vi "Accelerometer Config Pane.vi"(6 "_SubPanelMessages":refnum<notifier>, 9 "_myEmbeddedToFrameEvent":T6, 10 "_myEmbedded.Exit":refnum<user-event>, 11 "_Property Bundle":cluster{"Name":string, "Value":variant}[](array[cluster])) -> (1 "_Connection Informations":T1, 2 "_Scripter Input":T8)   [LabVIEW 2021]
doc: "Reads acceleration values along the X, Y, and Z axes of the accelerometer on the NI myRIO."
uses:
  <vilib>/myRIO/Common/Express VI Framework/typedefs/Config Pane to Framework Ref.ctl
  <vilib>/myRIO/Common/Express VI Framework/typedefs/Data Validate Ref.ctl
  <vilib>/myRIO/Common/Express VI Framework/typedefs/Scripter Input.ctl
  <vilib>/myRIO/Common/Express VI Framework/typedefs/WireThrough Terminal Names.ctl
  <vilib>/myRIO/Common/Express VI Framework/typedefs/Instrument Driver Method Descriptor Array.ctl
  <vilib>/myRIO/Common/Express VI Framework/typedefs/Instrument Driver Method Descriptor.ctl
  <vilib>/myRIO/Common/Express VI Framework/typedefs/Sub Panel Messages.ctl
  <vilib>/myRIO/Express VI/Onboard Devices/Accelerometer/Accelerometer Images.ctl
  <vilib>/myRIO/Common/Express VI Framework/typedefs/Connection Informations.ctl
  <vilib>/myRIO/Common/Instrument Driver Framework/Utilities/typedefs/Channel Types.ctl
  <vilib>/myRIO/Common/Express VI Framework/vis/Express VI Framework Strings Global.vi
panel:
  out "_AccelerometerAxes":T2
  in  "Z Axis Custom Terminal Name":string
  in  "Z Enable":bool=TRUE
  in  "Y Axis Custom Terminal Name":string
  in  "Y Enable":bool=TRUE
  in  "X Axis Custom Terminal Name":string
  in  "X Enable":bool=TRUE
  in  "_Default Alias String":string
  in  "_VI Default Name (Edit and make value default)":string="Accelerometer"
  in  "Name:":string caption="Node name:"
  in  "_WireThrough Info (Edit and make value default)":T3={"WireThrough Top In"="Accelerometer Ref In", "WireThrough Bottom In"="error in (no error)", "WireThrough Top Out"="Accelerometer Ref Out", "WireThrough Bottom Out"="error out"}
  in  "_Template Array (Edit and make value default)":T4=[{"Function Name"="Smart Open", "VI Path"=path "<vilib>/myRIO/Instrument Drivers/Onboard Devices/Accelerometer/vis", "Script"=TRUE, "Inputs"=[{"name"="Channel Names", "value"=variant, "Config Pane Only"=TRUE, "Build Array"=FALSE, "Bundle Cluster"=FALSE, "Show Term"=FALSE, "alias"=[], "Required Input"=FALSE}], "Outputs"=[], "VI Class"=enum."Open", "Controls Refs[]"=[], "Inline"=FALSE}, {"Function Name"="Open", "VI Path"=path "<vilib>/myRIO/Instrument Drivers/Onboard Devices/Accelerometer/vis", "Script"=FALSE, "Inputs"=[], "Outputs"=[{"name"="Values", "value"=variant, "Show Term"=TRUE, "Index Array"=TRUE, "Unbundle Cluster"=FALSE, "alias"=["AccelerationX", "AccelerationY", "AccelerationZ"]}], "VI Class"=enum."Open", "Controls Refs[]"=[], "Inline"=FALSE}, {"Function Name"="Read", "VI Path"=path "<vilib>/myRIO/Instrument Drivers/Onboard Devices/Accelerometer/vis", "Script"=TRUE, "Inputs"=[], "Outputs"=[{"name"="Values", "value"=variant, "Show Term"=TRUE, "Index Array"=TRUE, "Unbundle Cluster"=FALSE, "alias"=["AccelerationX", "AccelerationY", "AccelerationZ"]}], "VI Class"=enum."Data", "Controls Refs[]"=[], "Inline"=FALSE}, {"Function Name"="Close", "VI Path"=path "<vilib>/myRIO/Instrument Drivers/Onboard Devices/Accelerometer/vis", "Script"=FALSE, "Inputs"=[], "Outputs"=[], "VI Class"=enum."Close", "Controls Refs[]"=[], "Inline"=FALSE}]
  in  "_Test Close":bool
  # "Range determines the sensitivity of the accelerometer."
  # "User Visible Area"
  # "Enable:"
  # "Custom channel name:"
  # "NOTE: Tab Order has been set\nfor this Front Panel.\n\nSee Edit>>Set Tabbing Order...\n\nAll controls that are not visible at \nruntime are excluded from Tabbing order\n\nTo exlude a control from context\nhelp prefix its label text with a '-'"
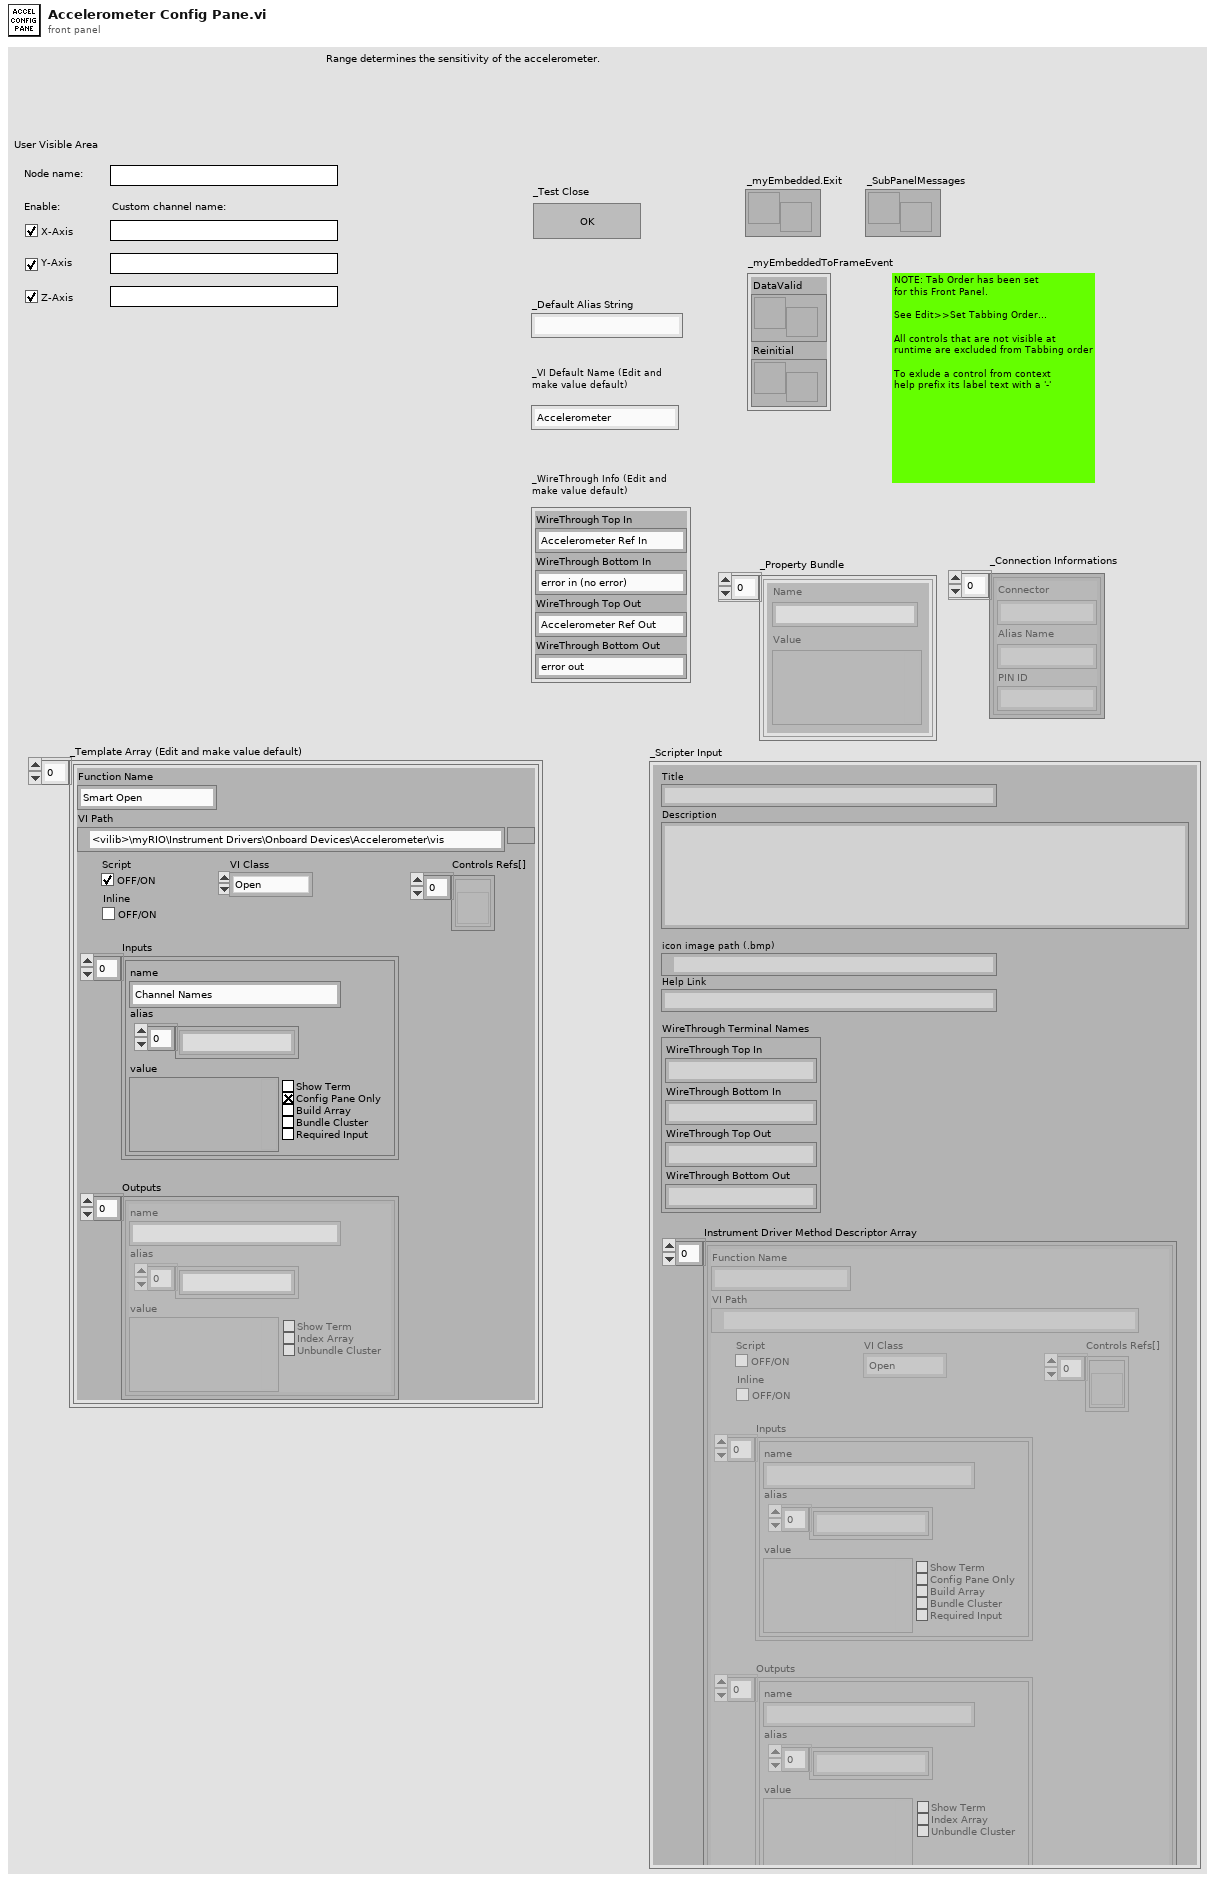
[diagram p1: front panel]
types:
  T1 = typedef "Connection Informations.ctl" = cluster{"Connector":string, "Alias Name":string, "PIN ID":string}[]
  T2 = typedef "Accelerometer Images.ctl" = u16
  T3 = typedef "WireThrough Terminal Names.ctl" = cluster{"WireThrough Top In":string, "WireThrough Bottom In":string, "WireThrough Top Out":string, "WireThrough Bottom Out":string}
  T4 = typedef "Instrument Driver Method Descriptor Array.ctl" = T5[]
  T5 = typedef "Instrument Driver Method Descriptor.ctl" = cluster{"Function Name":string, "VI Path":path, "Script":bool, "Inputs":cluster{"name":string, "value":variant, "Config Pane Only":bool, "Build Array":bool, "Bundle Cluster":bool, "Show Term":bool, "alias":string[], "Required Input":bool}[], "Outputs":cluster{"name":string, "value":variant, "Show Term":bool, "Index Array":bool, "Unbundle Cluster":bool, "alias":string[]}[], "VI Class":enum16{"Open", "Configure", "Data", "Manage", "Close"}, "Controls Refs[]":refnum<vi>[], "Inline":bool}
  T6 = typedef "Config Pane to Framework Ref.ctl" = cluster{"DataValid":T7, "Reinitial":refnum<user-event>}
  T7 = typedef "Data Validate Ref.ctl" = refnum<user-event>
  T8 = typedef "Scripter Input.ctl" = cluster{"Title":string, "Description":string, "icon image path (.bmp)":path, "Help Link":string, "WireThrough Terminal Names":T3, "Instrument Driver Method Descriptor Array":T4}
  T9 = enum8{"Enabled", "Disabled", "Disabled and Grayed Out"}
  T10 = typedef "Channel Types.ctl" = enum32{"Unknown", "AI", "AO", "DIO - DI", "DIO", "DIO - DO", "I2C", "PWM", "Encoder", "SPI", "UART", "Accelerometer", "DIO - LED", "DIO - Button", "AI (N Samples)", "AudioIn (N Samples)", "AO (N Samples)", "AudioOut (N Samples)", "DI (N Samples)", "DO (N Samples)", "AI IRQ", "DI IRQ", "Timer IRQ", "RSL", "Relay", "CAN", "AI (Continuous)", "AO (Continuous)"}
  T11 = typedef "Sub Panel Messages.ctl" = enum16{"Initialized"}
  T12 = typedef "Channel Info.ctl" = cluster{"Channel Name":string, "Alias":string, "Used?":bool, "Not Support?":bool, "Property Bundle":cluster{"Name":string, "Value":variant}[]}
  T13 = cluster{"name":string, "value":variant, "Config Pane Only":bool, "Build Array":bool, "Bundle Cluster":bool, "Show Term":bool, "alias":string[], "Required Input":bool}[]
  T14 = cluster{"name":string, "value":variant, "Config Pane Only":bool, "Build Array":bool, "Bundle Cluster":bool, "Show Term":bool, "alias":string[], "Required Input":bool}
  T15 = cluster{"name":string, "value":variant, "Show Term":bool, "Index Array":bool, "Unbundle Cluster":bool, "alias":string[]}[]
  T16 = cluster{"name":string, "value":variant, "Show Term":bool, "Index Array":bool, "Unbundle Cluster":bool, "alias":string[]}
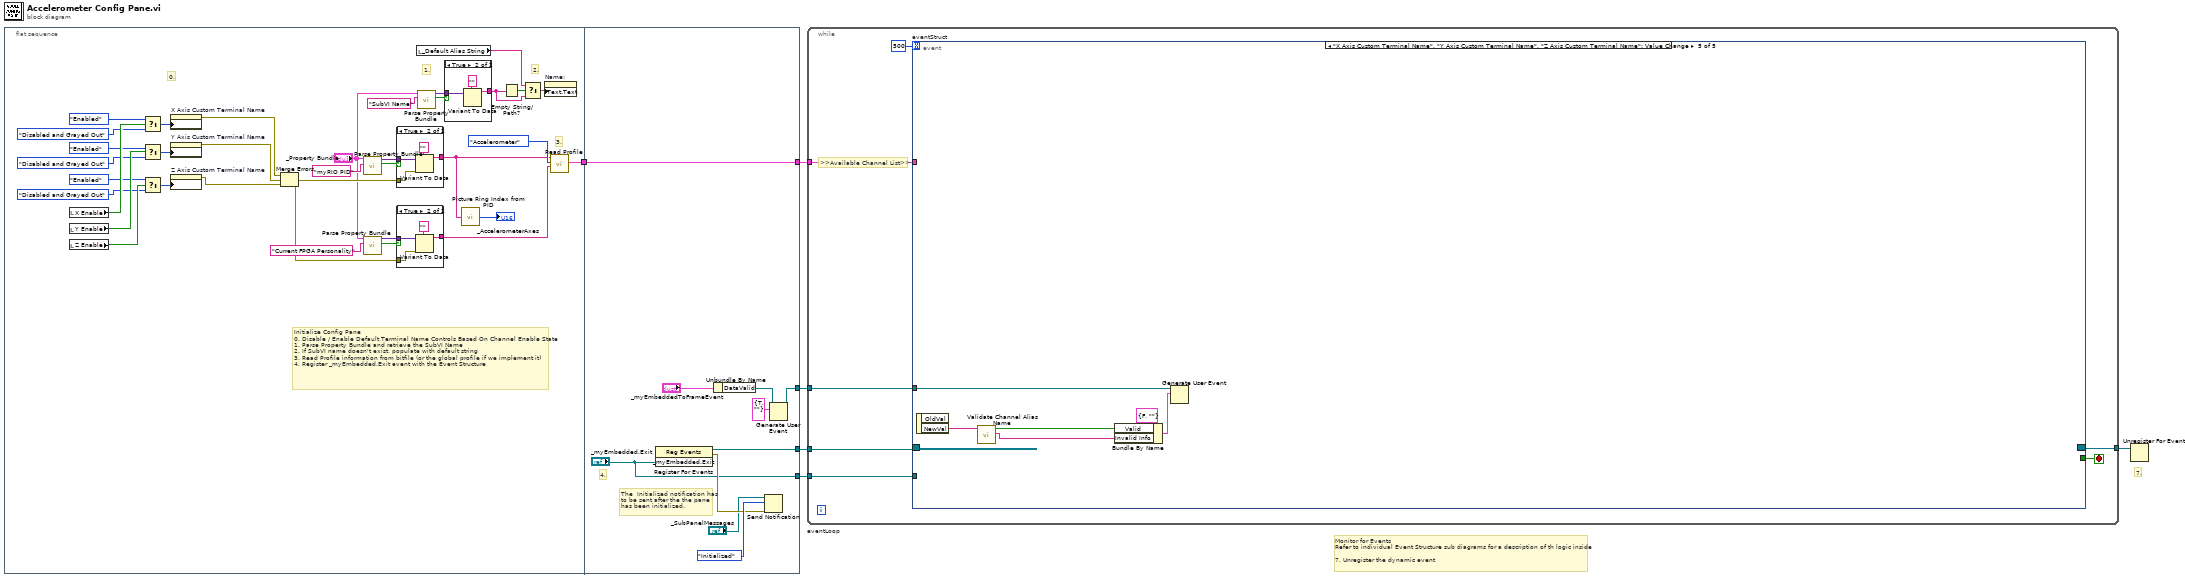
[diagram p0: block diagram]
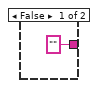
[diagram p2: hidden frame]
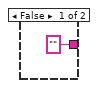
[diagram p3: hidden frame]
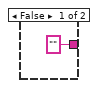
[diagram p4: hidden frame]
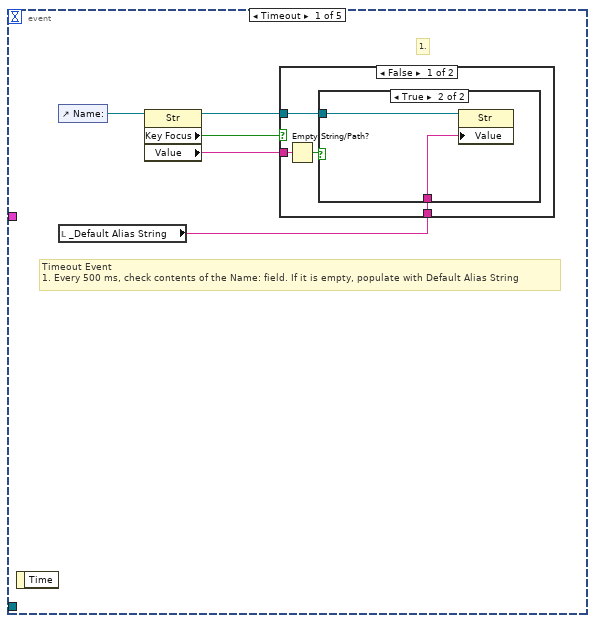
[diagram p5: hidden frame]
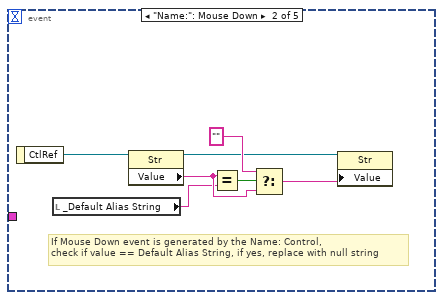
[diagram p8: hidden frame]
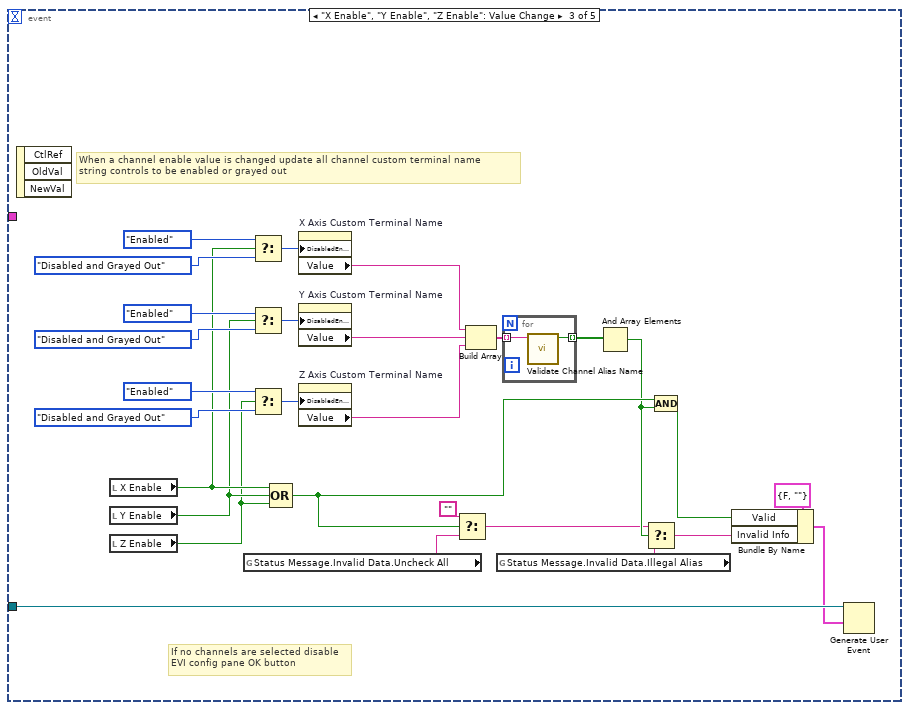
[diagram p9: hidden frame]
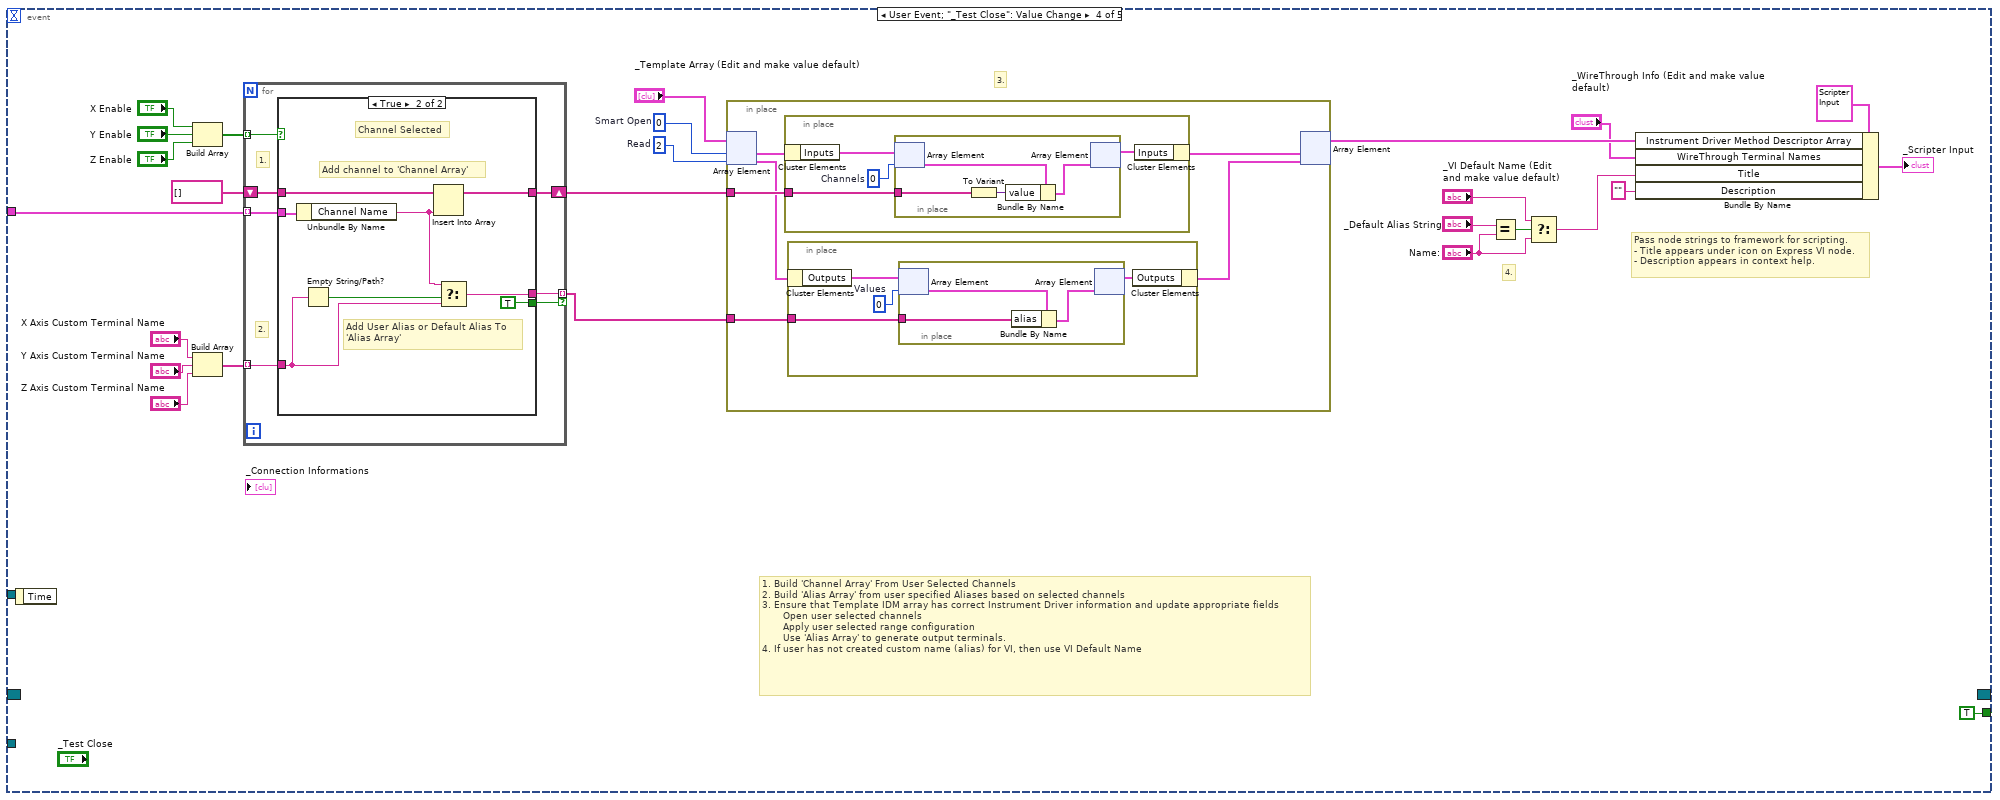
[diagram p10: hidden frame]
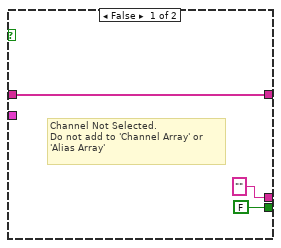
[diagram p11: hidden frame]
diagram:
  # "7."
  # "Monitor for Events\nRefer to individual Event Structure sub diagrams for a description of th logic inside\n\n7. Unregister the dynamic event"
  n1 = flat-sequence {
    tunnel: [w41] -> w4
    tunnel: [w65] -> w5
    tunnel: w4 -> [w65]
    tunnel: [w57] -> w3
    tunnel: [w60] -> w2
    tunnel: ["_myEmbedded.Exit"] -> w1
    frame #0 {
      # "Initialize Config Pane\n0. Disable / Enable Default Terminal Name Controls Based On Channel Enable State\n1. Parse Property Bundle and retrieve the SubVI Name\n2. If SubVI name doesn't exist, populate with default string\n3. Read Profile information from bitfile (or the global profile if we implement it)\n4. Register _myEmbedded.Exit event with the Event Structure"
      # "0."
      # "3."
      # "1."
      # "2."
      n2 = local read "X Enable"() -> (w28:bool)
      n3 = local read "Y Enable"() -> (w29:bool)
      n4 = local read "Z Enable"() -> (w30:bool)
      n5 = Select(t=T9."Enabled" ("Disabled"), s=w28, f=T9."Disabled and Grayed Out" ("Disabled")) -> (s? t:f=w27:T9)
      n6 = Select(t=T9."Enabled" ("Disabled"), s=w29, f=T9."Disabled and Grayed Out" ("Disabled")) -> (s? t:f=w24:T9)
      n7 = Select(t=T9."Enabled" ("Disabled"), s=w30, f=T9."Disabled and Grayed Out" ("Disabled")) -> (s? t:f=w23:T9)
      n8 = property on="X Axis Custom Terminal Name" class="Str"("DisabledEnum"=w27) -> (error out=w18:errorcluster)  [unwired: 2 in, 1 out]
      n9 = property on="Y Axis Custom Terminal Name" class="Str"("DisabledEnum"=w24) -> (error out=w17:errorcluster)  [unwired: 2 in, 1 out]
      n10 = property on="Z Axis Custom Terminal Name" class="Str"("DisabledEnum"=w23) -> (error out=w16:errorcluster)  [unwired: 2 in, 1 out]
      n11 = Merge Errors(w18, w17, w16) -> (w9:errorcluster)
      n12 = call <vilib>:"Parse Property Bundle.vi"("Name"="myRIO PID", "Property Bundle"="_Property Bundle") -> ("Found?"=w40:bool, "Value"=w39:variant)  [unwired: 8 in]
      n13 = call <vilib>:"Parse Property Bundle.vi"("Name"="Current FPGA Personality", "Property Bundle"="_Property Bundle") -> ("Found?"=w10:bool, "Value"=w11:variant)  [unwired: 8 in]
      n14 = case shown="True" w40 {
        tunnel: w39 -> [_ w55]
        tunnel: ["" ("Name") w53] -> w13
        tunnel: w9 -> [_ w52]
        frame False {
        }
        frame True {
          n15 = Variant To Data(error in=w52, type="" ("Name"), Variant=w55) -> (data=w53:string)  [unwired: 1 out]
        }
      }
      n16 = case shown="True" w10 {
        tunnel: w11 -> [_ w46]
        tunnel: ["" ("Name") w44] -> w8
        tunnel: w9 -> [_ w43]
        frame False {
        }
        frame True {
          n17 = Variant To Data(error in=w43, type="" ("Name"), Variant=w46) -> (data=w44:string)  [unwired: 1 out]
        }
      }
      n18 = local read "_Default Alias String"() -> (w35:string)
      n19 = call <vilib>:"Parse Property Bundle.vi"("Name"="SubVI Name", "Property Bundle"="_Property Bundle") -> ("Found?"=w33:bool, "Value"=w32:variant)  [unwired: 8 in]
      n20 = case shown="True" w33 {
        tunnel: w32 -> [_ w50]
        tunnel: ["" ("Name") w48] -> w31
        frame False {
        }
        frame True {
          n21 = Variant To Data(type="" ("Name"), Variant=w50) -> (data=w48:string)  [unwired: 1 in, 1 out]
        }
      }
      n22 = call <vilib>:"Picture Ring Index from PID.vi"("myRIO PID"=w13) -> ("picture ring index"=→"_AccelerometerAxes":u32)
      n23 = Empty String/Path?(string/path=w31) -> (empty?=w37:bool)
      n24 = Select(t=w35, s=w37, f=w31) -> (s? t:f=w36:string)
      n25 = property on="Name:" class="Str"("Text.Text"=w36) -> ()  [unwired: 2 in, 2 out]
      n26 = call <vilib>:"Read Profile.vi"("FPGA Name"=w8, "Channel to Read"=Channel_Types."Accelerometer", "myRIO PID"=w13) -> ("Channel List Out"=w41:T12[])  [unwired: 7 in, 1 out]
    }
    frame #1 {
      # "The  Initialized notification has to be sent after the the pane has been initialized."
      # "4."
      n27 = register-events("_myEmbedded.Exit") -> (reference out=w60:refnum<event-registration>, error out=w63:errorcluster)  [unwired: 2 in]
      n28 = Unbundle By Name("_myEmbeddedToFrameEvent") -> ("DataValid"=w58:T7)
      n29 = Send Notification(notification=Sub_Panel_Messages."Initialized", notifier="_SubPanelMessages", error in (no error)=w63) -> ()  [unwired: 2 out]
      n30 = Generate User Event(user event=w58, event data cluster=cluster{"Valid":bool, "Invalid Info":string} {"Valid"=TRUE, "Invalid Info"=""} ("event data")) -> (user event out=w57:T7)  [unwired: 2 in, 1 out]
    }
  }
  n31 = while "eventLoop" {
    tunnel: w2 -> [w71]
    tunnel: [w70] -> w6
    tunnel: w3 -> [w66]
    tunnel: w5 -> [w68]
    tunnel: w1 -> [w67]
    stop <- w72 stop-if-true
    # ">>Available Channel List>>"
    n32 = event "eventStruct" shown="[4] \"X Axis Custom Terminal Name\", \"Y Axis Custom Terminal Name\", \"Z Axis Custom Terminal Name\": Value Change" {
      selector: w71 -> [_ _ _ _ _]
      dyn-events: [_ _ _ _ _] -> w70
      timeout: 500 -> [_ _ _ _ _]
      tunnel: [_ _ _ TRUE ("_Test Close") _] -> w72
      tunnel: w68 -> [_ _ _ w129 _]
      tunnel: w67 -> [_ _ _ _ _]
      tunnel: w66 -> [_ _ w118 _ w188]
      event Timeout {
        # "Timeout Event\n1. Every 500 ms, check contents of the Name: field. If it is empty, populate with Default Alias String"
        # "1."
        n33 = event-data() -> ()  [unwired: 1 in, 1 out]
        n34 = control-ref of="Name:"() -> (w75:refnum<vi>)
        n35 = local read "_Default Alias String"() -> (w73:string)
        n36 = property on="Property Node" class="Str"(reference=w75) -> (reference out=w74:refnum<vi>, "Key Focus"=w76:bool, "Value"=w77:string)  [unwired: 1 in, 1 out]
        n37 = case shown="False" w76 {
          tunnel: w77 -> [w81 _]
          tunnel: w74 -> [w79 _]
          tunnel: w73 -> [w78 _]
          frame False {
            n38 = Empty String/Path?(string/path=w81) -> (empty?=w80:bool)
            n39 = case shown="True" w80 {
              tunnel: w79 -> [_ w83]
              tunnel: w78 -> [_ w82]
              frame False {
              }
              frame True {
                n40 = property on="Property Node" class="Str"(reference=w83, "Value"=w82) -> ()  [unwired: 1 in, 2 out]
              }
            }
          }
          frame True {
          }
        }
      }
      event "Name:": Mouse Down {
        # "If Mouse Down event is generated by the Name: Control,\ncheck if value == Default Alias String, if yes, replace with null string"
        n41 = event-data() -> ("CtlRef"=w90:refnum<vi>)  [unwired: 1 in]
        n42 = local read "_Default Alias String"() -> (w84:string)
        n43 = property class="Str"(reference=w90) -> (reference out=w86:refnum<vi>, "Value"=w85:string)  [unwired: 1 in, 1 out]
        n44 = Equal?(x=w85, y=w84) -> (x = y?=w89:bool)
        n45 = Select(t="", s=w89, f=w85) -> (s? t:f=w87:string)
        n46 = property class="Str"(reference=w86, "Value"=w87) -> ()  [unwired: 1 in, 2 out]
      }
      event "X Enable", "Y Enable", "Z Enable": Value Change {
        # "When a channel enable value is changed update all channel custom terminal name \nstring controls to be enabled or grayed out"
        # "If no channels are selected disable\nEVI config pane OK button"
        n47 = event-data() -> ()  [unwired: 1 in, 3 out]
        n48 = local read "X Enable"() -> (w108:bool)
        n49 = local read "Y Enable"() -> (w107:bool)
        n50 = local read "Z Enable"() -> (w106:bool)
        n51 = global read "Express VI Framework Strings Global.vi" "Status Message.Invalid Data.Uncheck All"() -> (w95:string)
        n52 = Select(t=T9."Enabled" ("Disabled"), s=w108, f=T9."Disabled and Grayed Out" ("Disabled")) -> (s? t:f=w109:T9)
        n53 = Select(t=T9."Enabled" ("Disabled"), s=w107, f=T9."Disabled and Grayed Out" ("Disabled")) -> (s? t:f=w112:T9)
        n54 = Select(t=T9."Enabled" ("Disabled"), s=w106, f=T9."Disabled and Grayed Out" ("Disabled")) -> (s? t:f=w113:T9)
        n55 = Compound Arithmetic op=OR(w108, w107, w106) -> (w97:bool)
        n56 = property on="X Axis Custom Terminal Name" class="Str"("DisabledEnum"=w109) -> ("Value"=w103:string)  [unwired: 2 in, 2 out]
        n57 = property on="Y Axis Custom Terminal Name" class="Str"("DisabledEnum"=w112) -> ("Value"=w102:string)  [unwired: 2 in, 2 out]
        n58 = property on="Z Axis Custom Terminal Name" class="Str"("DisabledEnum"=w113) -> ("Value"=w101:string)  [unwired: 2 in, 2 out]
        n59 = Select(t="", s=w97, f=w95) -> (s? t:f=w93:string)
        n60 = Build Array(w103, w102, w101) -> (w100:string[])
        n61 = global read "Express VI Framework Strings Global.vi" "Status Message.Invalid Data.Illegal Alias"() -> (w92:string)
        n62 = for {
          tunnel: w100 -> [w120] mode=indexing
          tunnel: [w119] -> w99 mode=indexing
          n63 = call <vilib>:"Validate Channel Alias Name.vi"("Channel Alias"=w120) -> ("Valid?"=w119:bool)  [unwired: 9 in, 1 out]
        }
        n64 = And Array Elements(Boolean array=w99) -> (logical AND=w94:bool)
        n65 = Select(t=w93, s=w94, f=w92) -> (s? t:f=w91:string)
        n66 = Compound Arithmetic op=AND(w97, w94) -> (w98:bool)
        n67 = Bundle By Name(cluster=cluster{"Valid":bool, "Invalid Info":string} {"Valid"=FALSE, "Invalid Info"=""} ("event data"), "Valid"=w98, "Invalid Info"=w91) -> (w104:cluster{"Valid":bool, "Invalid Info":string})
        n68 = Generate User Event(user event=w118, event data cluster=w104) -> ()  [unwired: 2 in, 2 out]
      }
      event User Event; "_Test Close": Value Change {
        w126 = 2  # Read
        w143 = 0  # Smart Open
        # "3."
        # "1. Build 'Channel Array' From User Selected Channels\n2. Build 'Alias Array' from user specified Aliases based on selected channels \n3. Ensure that Template IDM array has correct Instrument Driver information and update appropriate fields\n       Open user selected channels\n       Apply user selected range configuration\n       Use 'Alias Array' to generate output terminals. \n4. If user has not created custom name (alias) for VI, then use VI Default Name"
        # "4."
        # "Pass node strings to framework for scripting.\n- Title appears under icon on Express VI node.\n- Description appears in context help."
        n69 = event-data() -> ()  [unwired: 1 in, 1 out]
        n70 = Build Array("X Enable", "Y Enable", "Z Enable") -> (w130:bool[])
        n71 = Build Array("X Axis Custom Terminal Name", "Y Axis Custom Terminal Name", "Z Axis Custom Terminal Name") -> (w121:string[])
        n72 = for {
          tunnel: w130 -> [w153] mode=indexing
          tunnel: w129 -> [w151] mode=indexing
          shift-right: [w150] -> w127
          shift-left: string[] [] ("array") -> [w152]
          tunnel: w121 -> [w148] mode=indexing
          tunnel: [w149] -> w125 mode=indexing if=w147
          # "2."
          # "1."
          n73 = case shown="True" w153 {
            tunnel: w152 -> [w156 w164]
            tunnel: w151 -> [_ w163]
            tunnel: [w156 w162] -> w150
            tunnel: ["" ("Z Axis Custom Terminal Name") w160] -> w149
            tunnel: w148 -> [_ w159]
            tunnel: [FALSE TRUE] -> w147
            frame False {
              # "Channel Not Selected.\nDo not add to 'Channel Array' or \n'Alias Array'"
            }
            frame True {
              # "Add User Alias or Default Alias To \n'Alias Array'"
              # "Add channel to 'Channel Array'"
              # "Channel Selected"
              n74 = Unbundle By Name(w163) -> ("Channel Name"=w157:string)
              n75 = Empty String/Path?(string/path=w159) -> (empty?=w161:bool)
              n76 = Insert Into Array(array=w164, new element=w157) -> (w162:string[])  [unwired: 1 in]
              n77 = Select(t=w157, s=w161, f=w159) -> (s? t:f=w160:string)
            }
          }
        }
        n78 = in-place {
          in-place-border: w127 -> [w168]
          in-place-border: w125 -> [w167]
          n79 = in-place-array #1("_Template Array (Edit and make value default)", w143, w126) -> (w170:T5, w166:T5)
          n80 = in-place {
            in-place-border: w168 -> [w180]
            w178 = 0  # Channels
            n81 = in-place-cluster #2(w170) -> ("Inputs"=w181:T13)
            n82 = in-place {
              in-place-border: w180 -> [w182]
              n83 = in-place-array #3(w181, w178) -> (w185:T14)
              n84 = To Variant(anything=w182) -> (Variant=w183:variant)
              n85 = Bundle By Name(cluster=w185, "value"=w183) -> (w184:T14)
              n86 = in-place-array #3(w184) -> (w179:T13)  [unwired: 1 out]
            }
            n87 = in-place-cluster #2("Inputs"=w179) -> (w169:T5)
          }
          n88 = in-place {
            in-place-border: w167 -> [w171]
            w174 = 0  # Values
            n89 = in-place-cluster #4(w166) -> ("Outputs"=w173:T15)
            n90 = in-place {
              in-place-border: w171 -> [w175]
              n91 = in-place-array #5(w173, w174) -> (w177:T16)
              n92 = Bundle By Name(cluster=w177, "alias"=w175) -> (w176:T16)
              n93 = in-place-array #5(w176) -> (w172:T15)  [unwired: 1 out]
            }
            n94 = in-place-cluster #4("Outputs"=w172) -> (w165:T5)
          }
          n95 = in-place-array #1(w169, w165) -> (w145:T4)  [unwired: 2 out]
        }
        n96 = Equal?(x="_Default Alias String", y="Name:") -> (x = y?=w137:bool)
        n97 = Select(t="_VI Default Name (Edit and make value default)", s=w137, f="Name:") -> (s? t:f=w136:string)
        n98 = Bundle By Name(cluster=T8 {"Title"="", "Description"="", "icon image path (.bmp)"=path "", "Help Link"="", "WireThrough Terminal Names"={"WireThrough Top In"="", "WireThrough Bottom In"="", "WireThrough Top Out"="", "WireThrough Bottom Out"=""}, "Instrument Driver Method Descriptor Array"=[]} ("Scripter Input"), "Instrument Driver Method Descriptor Array"=w145, "WireThrough Terminal Names"="_WireThrough Info (Edit and make value default)", "Title"=w136, "Description"="" ("Title")) -> (→"_Scripter Input":T8)
      }
      event "X Axis Custom Terminal Name", "Y Axis Custom Terminal Name", "Z Axis Custom Terminal Name": Value Change {
        n99 = event-data() -> ("NewVal"=w191:string)  [unwired: 1 in, 1 out]
        n100 = call <vilib>:"Validate Channel Alias Name.vi"("Channel Alias"=w191) -> ("Invalid Info"=w186:string, "Valid?"=w187:bool)  [unwired: 9 in]
        n101 = Bundle By Name(cluster=cluster{"Valid":bool, "Invalid Info":string} {"Valid"=FALSE, "Invalid Info"=""} ("event data"), "Valid"=w187, "Invalid Info"=w186) -> (w189:cluster{"Valid":bool, "Invalid Info":string})
        n102 = Generate User Event(user event=w188, event data cluster=w189) -> ()  [unwired: 2 in, 2 out]
      }
    }
  }
  n103 = Unregister For Events(event registration refnum=w6) -> ()  [unwired: 1 in, 1 out]
